vi "General_ErrorHandler.vi"(6 "error in":errorcluster, 8 "Prev Master State Input":T1=enum."Init") -> (0 "error out":errorcluster, 3 "All-Quit":bool, 5 "Next State":T1=enum."Init")   [LabVIEW 2021]
doc: "Resets the CCD camera controller and initializes it with Setup String. The default Setup String is \"ldb,1,16,u,0,225,25,b,1,15;sdu,0,1024,1024;cl0;omrm;sron\". \nError, if no -1, is set as 0 if a serial poll detects an error (bit 15 in status bit set)\n\nSet the CCD Setup String Global variable after the command is complete."
uses:
  LV7/OpticsSS.ctl
  <vilib>/Utility/error.llb/DialogType.ctl
  Globals and TypeDefs/Type Definitions.llb/3 way Status.ctl
  Globals and TypeDefs/gDetector.vi
  Globals and TypeDefs/gSpectrometer.vi
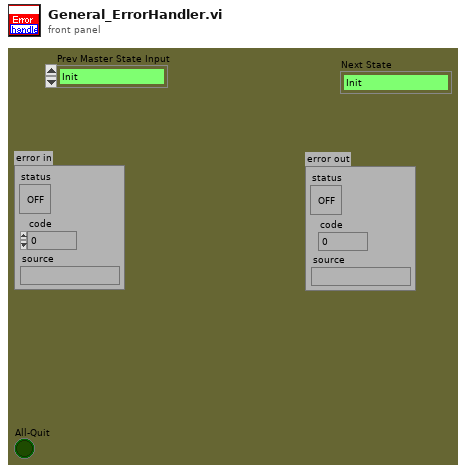
[diagram p1: front panel]
types:
  T1 = typedef "OpticsSS.ctl" = enum16{"_Quit_", "Init", "Ready", "HTL", "CCD_shot", "QueueData", "Error Handler", "HTL Error", "CCD Error", "CCDSetup", "Calibration", "BG_Setup", "HTL Paras Setup"}
  T2 = enum16{"--Quit--", "Init GPIB", "Poll GPIB", "Wait for SRQ", "Clear CCD Parameters", "New CCD Parameters", "Check CCD Command Error"}
  T3 = enum16{"End", "Init", "Reset", "SetAcqParameter", "SetArea", "Start Acquisition", "Busy Status Poll", "Read", "Stop"}
  T4 = typedef "DialogType.ctl" = u16
  T5 = typedef "Error Categories.ctt" = enum8{"General", "CCD-256x1024", "CCD-1340x400", "InGaAs PDA", "McPherson 2075", "Magnetic Field", "Temperature Control", "Other"}
  T6 = enum16{"Left Button", "Center Button", "Right Button", "Window Close"}
  T7 = typedef "3 way Status.ctl" = u8
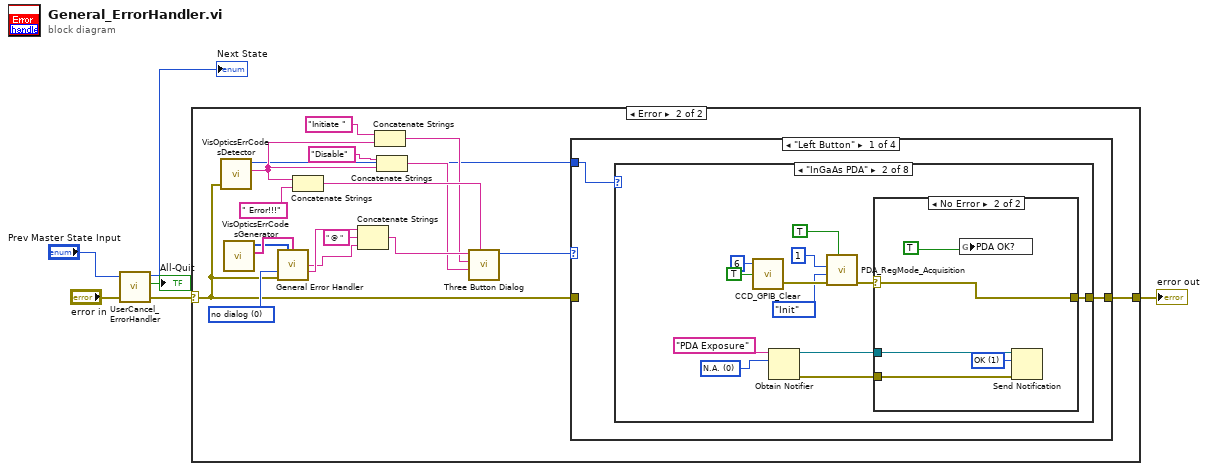
[diagram p0: block diagram]
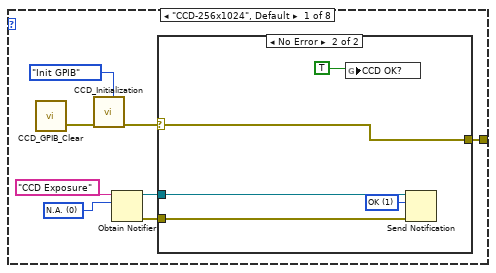
[diagram p3: hidden frame]
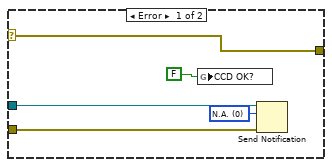
[diagram p4: hidden frame]
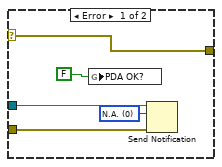
[diagram p5: hidden frame]
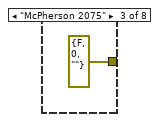
[diagram p6: hidden frame]
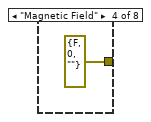
[diagram p7: hidden frame]
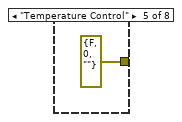
[diagram p8: hidden frame]
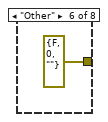
[diagram p9: hidden frame]
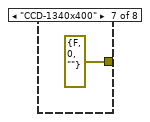
[diagram p10: hidden frame]
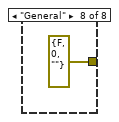
[diagram p11: hidden frame]
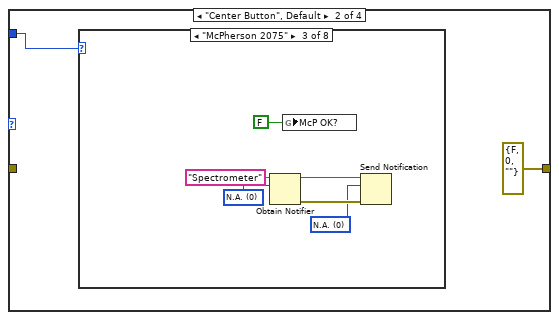
[diagram p12: hidden frame]
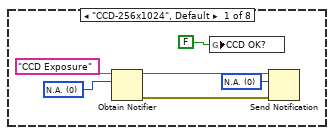
[diagram p13: hidden frame]
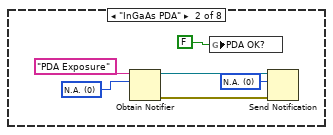
[diagram p14: hidden frame]
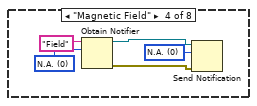
[diagram p15: hidden frame]
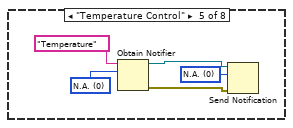
[diagram p16: hidden frame]
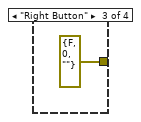
[diagram p20: hidden frame]
diagram:
  n1 = call "UserCancel_ErrorHandler.vi"("error in"="error in", "Prev Master State Input"="Prev Master State Input") -> ("error out"=w5:errorcluster, "All-Quit"=→"All-Quit":bool, "Next State"=→"Next State":T1)  [unwired: 4 in]
  n2 = case shown="Error" w5 {
    selector: w5 -> [w7 w20]
    tunnel: [w7 w21] -> w6
    frame No Error {
    }
    frame Error {
      w23 = T4 0 items=["no dialog", "OK message", "continue or stop message", "OK message + warnings", "continue/stop + warnings"] ("type of dialog (OK msg:1)")
      n3 = call "VisOpticsErrCodesDetector.vi"("error in"=w20) -> ("NHMFL Visible Optics Error Category"=w8:T5, "Error Category text"=w10:string)  [unwired: 2 in, 2 out]
      n4 = call "VisOpticsErrCodesGenerator.vi"() -> ("user-defined descriptions"=w25:string[], "user-defined codes"=w24:i32[])  [unwired: 3 in, 4 out]
      n5 = call <vilib>:"General Error Handler.vi"("[user-defined codes]"=w24, "[user-defined descriptions]"=w25, "type of dialog (OK msg:1)"=w23, "error in (no error)"=w20) -> ("source out"=w15:string, "message"=w17:string)  [unwired: 7 in, 3 out]
      n6 = Concatenate Strings(w10, " Error!!!" ("string")) -> (w18:string)
      n7 = Concatenate Strings(w17, " @ " ("string"), w15) -> (w14:string)
      n8 = Concatenate Strings("Initiate " ("Left Button Text (\"Yes\")"), w10) -> (w12:string)
      n9 = Concatenate Strings("Disable" ("Center Button Text (\"No\")"), w10) -> (w9:string)
      n10 = call <vilib>:"Three Button Dialog.vi"("Window Title (\"\")"=w18, "Center Button Text (\"No\")"=w9, "Left Button Text (\"Yes\")"=w12, "message"=w14) -> ("Which Button?"=w22:T6)  [unwired: 7 in]
      n11 = case shown="\"Left Button\"" w22 {
        tunnel: [w27 errorcluster {"status"=FALSE, "code"=0, "source"=""} ("error IO") errorcluster {"status"=FALSE, "code"=0, "source"=""} ("error IO") errorcluster {"status"=FALSE, "code"=0, "source"=""} ("error IO")] -> w21
        tunnel: w20 -> [_ _ _ _]
        tunnel: w8 -> [w26 w74 _ _]
        frame "Left Button" {
          n12 = case shown="\"InGaAs PDA\"" w26 {
            tunnel: [w32 w55 errorcluster {"status"=FALSE, "code"=0, "source"=""} ("error IO") errorcluster {"status"=FALSE, "code"=0, "source"=""} ("error IO") errorcluster {"status"=FALSE, "code"=0, "source"=""} ("error IO") errorcluster {"status"=FALSE, "code"=0, "source"=""} ("error IO") errorcluster {"status"=FALSE, "code"=0, "source"=""} ("error IO") errorcluster {"status"=FALSE, "code"=0, "source"=""} ("error IO")] -> w27
            frame "CCD-256x1024", Default {
              w28 = T7 0 items=["N.A.", "OK", "Busy", "Done"] ("H(T)")
              n13 = call "CCD_GPIB_Clear.vi"() -> ("error out"=w34:errorcluster)  [unwired: 5 in]
              n14 = call "CCD_Initialization.vi"("error in"=w34, "Starting Action"=T2."Init GPIB") -> ("error out"=w33:errorcluster)  [unwired: 3 in, 4 out]
              n15 = Obtain Notifier(name (unnamed)="CCD Exposure", notification data type=w28) -> (notifier out=w30:refnum<notifier>, error out=w29:errorcluster)  [unwired: 2 in, 1 out]
              n16 = case shown="No Error" w33 {
                selector: w33 -> [w38 w41]
                tunnel: w30 -> [w37 w43]
                tunnel: w29 -> [w36 w42]
                tunnel: [w38 w41] -> w32
                frame Error {
                  w40 = T7 0 items=["N.A.", "OK", "Busy", "Done"] ("notification")
                  n17 = global write "gDetector.vi" "CCD OK?"(FALSE ("CCD OK?")) -> ()
                  n18 = Send Notification(notification=w40, notifier=w37, error in (no error)=w36) -> ()  [unwired: 2 out]
                }
                frame No Error {
                  w45 = T7 1 items=["N.A.", "OK", "Busy", "Done"] ("notification")
                  n19 = global write "gDetector.vi" "CCD OK?"(TRUE ("CCD OK?")) -> ()
                  n20 = Send Notification(notification=w45, notifier=w43, error in (no error)=w42) -> ()  [unwired: 2 out]
                }
              }
            }
            frame "InGaAs PDA" {
              w48 = T7 0 items=["N.A.", "OK", "Busy", "Done"] ("H(T)")
              n21 = call "CCD_GPIB_Clear.vi"("Device Clear?"=TRUE, "GPIB Address"=i16 6) -> ("error out"=w57:errorcluster)  [unwired: 3 in]
              n22 = Obtain Notifier(name (unnamed)="PDA Exposure", notification data type=w48) -> (notifier out=w47:refnum<notifier>, error out=w46:errorcluster)  [unwired: 2 in, 1 out]
              n23 = call "PDA_RegMode_Acquisition.vi"("Shutter"=TRUE, "error in"=w57, "StartIng Mode"=T3."Init", "Number of Cycles"=u32 1) -> ("error out"=w56:errorcluster)  [unwired: 1 in, 3 out]
              n24 = case shown="No Error" w56 {
                selector: w56 -> [w58 w63]
                tunnel: w47 -> [w60 w65]
                tunnel: w46 -> [w59 w64]
                tunnel: [w58 w63] -> w55
                frame Error {
                  w62 = T7 0 items=["N.A.", "OK", "Busy", "Done"] ("notification")
                  n25 = global write "gDetector.vi" "PDA OK?"(FALSE ("CCD OK?")) -> ()
                  n26 = Send Notification(notification=w62, notifier=w60, error in (no error)=w59) -> ()  [unwired: 2 out]
                }
                frame No Error {
                  w67 = T7 1 items=["N.A.", "OK", "Busy", "Done"] ("notification")
                  n27 = global write "gDetector.vi" "PDA OK?"(TRUE ("CCD OK?")) -> ()
                  n28 = Send Notification(notification=w67, notifier=w65, error in (no error)=w64) -> ()  [unwired: 2 out]
                }
              }
            }
            frame "McPherson 2075" {
            }
            frame "Magnetic Field" {
            }
            frame "Temperature Control" {
            }
            frame "Other" {
            }
            frame "CCD-1340x400" {
            }
            frame "General" {
            }
          }
        }
        frame "Center Button", Default {
          n29 = case shown="\"McPherson 2075\"" w74 {
            frame "CCD-256x1024", Default {
              w77 = T7 0 items=["N.A.", "OK", "Busy", "Done"] ("notification")
              w78 = T7 0 items=["N.A.", "OK", "Busy", "Done"] ("H(T)")
              n30 = Obtain Notifier(name (unnamed)="CCD Exposure", notification data type=w78) -> (notifier out=w80:refnum<notifier>, error out=w79:errorcluster)  [unwired: 2 in, 1 out]
              n31 = global write "gDetector.vi" "CCD OK?"(FALSE ("CCD OK?")) -> ()
              n32 = Send Notification(notification=w77, notifier=w80, error in (no error)=w79) -> ()  [unwired: 2 out]
            }
            frame "InGaAs PDA" {
              w83 = T7 0 items=["N.A.", "OK", "Busy", "Done"] ("notification")
              w86 = T7 0 items=["N.A.", "OK", "Busy", "Done"] ("H(T)")
              n33 = Obtain Notifier(name (unnamed)="PDA Exposure", notification data type=w86) -> (notifier out=w85:refnum<notifier>, error out=w84:errorcluster)  [unwired: 2 in, 1 out]
              n34 = global write "gDetector.vi" "PDA OK?"(FALSE ("CCD OK?")) -> ()
              n35 = Send Notification(notification=w83, notifier=w85, error in (no error)=w84) -> ()  [unwired: 2 out]
            }
            frame "McPherson 2075" {
              w89 = T7 0 items=["N.A.", "OK", "Busy", "Done"] ("notification")
              w92 = T7 0 items=["N.A.", "OK", "Busy", "Done"] ("Saving")
              n36 = Obtain Notifier(name (unnamed)="Spectrometer", notification data type=w92) -> (notifier out=w91:refnum<notifier>, error out=w90:errorcluster)  [unwired: 2 in, 1 out]
              n37 = global write "gSpectrometer.vi" "McP OK?"(FALSE ("McP OK?")) -> ()
              n38 = Send Notification(notification=w89, notifier=w91, error in (no error)=w90) -> ()  [unwired: 2 out]
            }
            frame "Magnetic Field" {
              w96 = T7 0 items=["N.A.", "OK", "Busy", "Done"] ("notification")
              w97 = T7 0 items=["N.A.", "OK", "Busy", "Done"] ("Saving")
              n39 = Obtain Notifier(name (unnamed)="Field", notification data type=w97) -> (notifier out=w95:refnum<notifier>, error out=w94:errorcluster)  [unwired: 2 in, 1 out]
              n40 = Send Notification(notification=w96, notifier=w95, error in (no error)=w94) -> ()  [unwired: 2 out]
            }
            frame "Temperature Control" {
              w101 = T7 0 items=["N.A.", "OK", "Busy", "Done"] ("notification")
              w102 = T7 0 items=["N.A.", "OK", "Busy", "Done"] ("Saving")
              n41 = Obtain Notifier(name (unnamed)="Temperature", notification data type=w102) -> (notifier out=w100:refnum<notifier>, error out=w99:errorcluster)  [unwired: 2 in, 1 out]
              n42 = Send Notification(notification=w101, notifier=w100, error in (no error)=w99) -> ()  [unwired: 2 out]
            }
            frame "Other" {
            }
            frame "CCD-1340x400" {
            }
            frame "General" {
            }
          }
        }
        frame "Right Button" {
        }
        frame "Window Close" {
        }
      }
    }
  }
  "error out" <- w6
